vi "update.vi"(6 "call chain index (1)":i32=1, 7 "vi ref (caller)":refnum<vi>, 8 "error in (no error)":errorcluster, 11 "status":string) -> (0 "error out":errorcluster)   [LabVIEW 2024, in "status manager.lvlib"]
uses:
  status manager.lvlib
  <vilib>/Hampel Software Engineering/Git API/Git API/SubVIs/GIT-8601 UTC Date-Time String.vi
  <vilib>/Hampel Software Engineering/HSE Logger/DEBUG.vi
  <vilib>/Hampel Software Engineering/HSE Logger/ERROR.vi
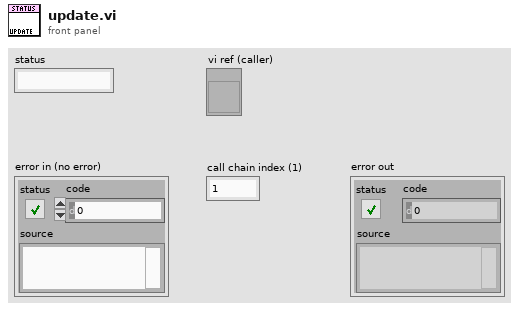
[diagram p1: front panel]
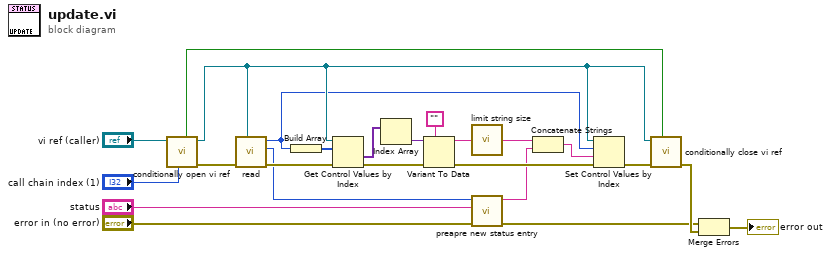
[diagram p0: block diagram]
diagram:
  n1 = call "conditionally open vi ref.vi"("call chain index (1)"="call chain index (1)", "vi ref in"="vi ref (caller)") -> ("error out"=w12:errorcluster, "vi ref out"=w9:refnum<vi>, "new ref?"=w8:bool)  [unwired: 7 in]
  n2 = call "read.vi"("vi ref (caller)"=w9, "error in (no error)"=w12) -> ("error out"=w24:errorcluster, "module id"=w3:i32, "status control id"=w2:i32)  [unwired: 7 in]
  n3 = Build Array(w2) -> (w18:i32[])
  n4 = Get Control Values by Index(0:w9, 1:w18, 3:w24) -> (10:w17:variant[], 11:w23:errorcluster)
  n5 = Index Array(array=w17) -> (element=w16:variant)  [unwired: 1 in]
  n6 = Variant To Data(error in=w23, type="", Variant=w16) -> (data=w14:string, error out=w22:errorcluster)
  n7 = call "limit string size.vi"("string in"=w14) -> ("string out"=w21:string)  [unwired: 1 in]
  n8 = call "preapre new status entry.vi"("error in (no error)"="error in (no error)", "new content"="status", "module id"=w3) -> ("error out"=w5:errorcluster, "new entry"=w19:string)  [unwired: 7 in]
  n9 = Concatenate Strings(w21, w19) -> (w13:string)
  n10 = Set Control Values by Index(0:w9, 1:w2, 2:w13, 3:w22) -> (11:w10:errorcluster)
  n11 = call "conditionally close vi ref.vi"("new ref?"=w8, "error in (no error)"=w10, "vi ref"=w9) -> ("error out"=w6:errorcluster)  [unwired: 8 in]
  n12 = Merge Errors(w5, w6) -> (→"error out":errorcluster)
